vi "configure.vi"(8 "error in (no error)":errorcluster, 9 "Value":i32, 10 "ILC":refnum<class "ILC.lvclass">, 11 "ConfigureILCDOStrategy in":refnum<class "ConfigureILCDOStrategy.lvclass">) -> (0 "error out":errorcluster, 2 "ILC 2":refnum<class "ILC.lvclass">, 3 "ConfigureILCDOStrategy out":refnum<class "ConfigureILCDOStrategy.lvclass">)   [LabVIEW 2015, in "ConfigureILCDOStrategy.lvclass"]
uses:
  ConfigureILCDOStrategy.lvclass
  <userlib>/Common/ILC/ILC/ILC.lvclass
  ConfigureILCDOStrategy.lvclass/ConfigureILCDOStrategy.ctl
  <userlib>/Common/ILC/ILC/ILC.lvclass/ILC.ctl
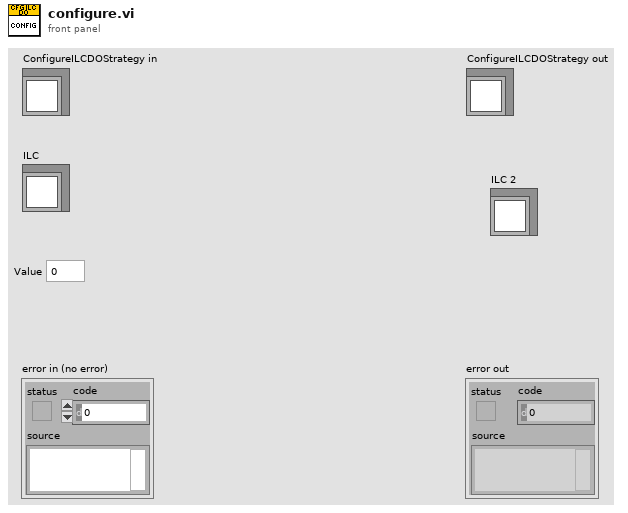
[diagram p1: front panel]
types:
  T1 = typedef "ILCBTTypedefs.lvlib/MUX Signals.ctl" = cluster{"MUX_A0 DAQ Channel to Write":refnum<k21>, "MUX_A1 DAQ Channel to Write":refnum<k21>}
  T2 = typedef "ILCBTTypedefs.lvlib/MUX Settings.ctl" = cluster{"MUX_AO":T3, "MUX_A1":T3}
  T3 = typedef "ILCBTTypedefs.lvlib/Digital Signal Level.ctl" = enum16{"Low", "High"}
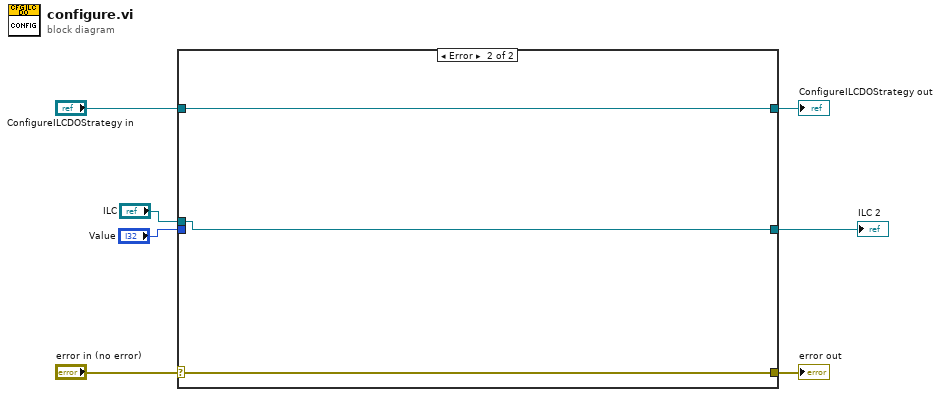
[diagram p0: block diagram]
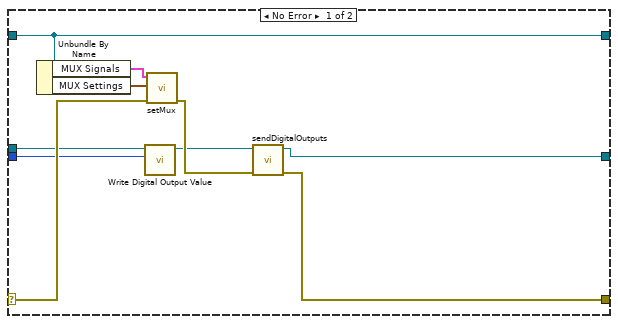
[diagram p2: hidden frame]
diagram:
  n1 = case shown="Error" "error in (no error)" {
    selector: "error in (no error)" -> [w14 w20]
    tunnel: [w13 w20] -> w6
    tunnel: [w17 w19] -> w4
    tunnel: "ConfigureILCDOStrategy in" -> [w17 w19]
    tunnel: "ILC" -> [w11 w18]
    tunnel: "Value" -> [w10 _]
    tunnel: [w8 w18] -> w1
    frame No Error {
      n2 = Unbundle By Name(w17) -> ("MUX Signals"=w16:T1, "MUX Settings"=w12:T2)
      n3 = call <userlib>:"Write Digital Output Value.vi"("Digital Output Value"=w10, "ILC in"=w11) -> ("ILC out"=w9:refnum<class "ILC.lvclass">)  [unwired: 9 in]
      n4 = call "setMux.vi"("error in (no error)"=w14, "MUX Settings"=w12, "MUX Signals"=w16) -> ("error out"=w15:errorcluster)  [unwired: 8 in]
      n5 = call <userlib>:"sendDigitalOutputs.vi"("error in (no error)"=w15, "ILC in"=w9) -> ("error out"=w13:errorcluster, "ILC out"=w8:refnum<class "ILC.lvclass">)  [unwired: 8 in]
    }
    frame Error {
    }
  }
  "error out" <- w6
  "ConfigureILCDOStrategy out" <- w4
  "ILC 2" <- w1
